vi "SetEnvTemp.vi"(11 "New temperature":dbl format="%.1f") -> (3 "Probe 1 temperature":dbl format="%.2f")   [LabVIEW 2009]
panel:
  out "error out":errorcluster
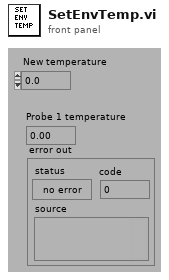
[diagram p1: front panel]
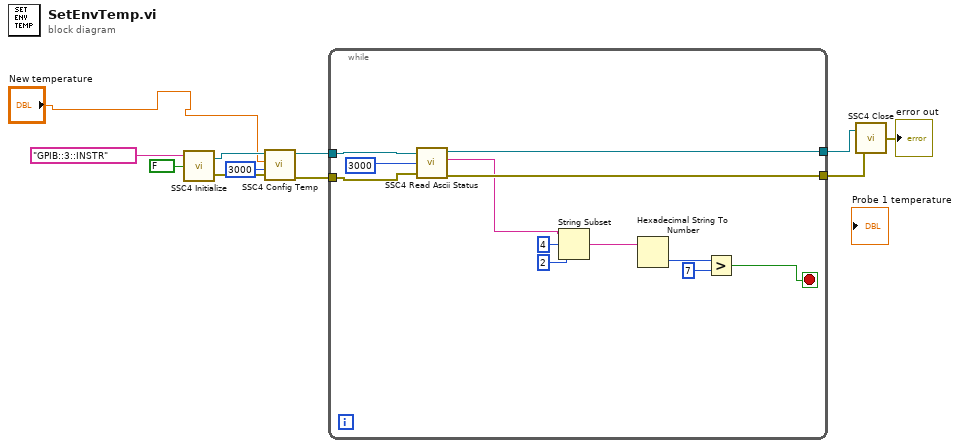
[diagram p0: block diagram]
diagram:
  n1 = call "SSC4 Initialize.vi"("reset"=FALSE, "instrument descriptor"="GPIB::3::INSTR") -> ("error out"=w8:errorcluster, "VISA session"=w9:refnum<visa-resource-name>)  [unwired: 1 in]
  n2 = call "SSC4 Config Temp.vi"("error in (no error)"=w8, "Command Delay"=u32 3000, "New temperature"="New temperature", "Visa Session"=w9) -> ("error out"=w5:errorcluster, "Dup Visa Session"=w6:refnum<visa-resource-name>)  [unwired: 6 in]
  n3 = while {
    tunnel: w6 -> [w23]
    tunnel: w5 -> [w22]
    tunnel: [w20] -> w3
    tunnel: [w19] -> w2
    stop <- w13 stop-if-true
    n4 = call "SSC4 Read Ascii Status.vi"("error in (no error)"=w22, "Command Delay (ms)"=u32 3000, "Visa Session"=w23) -> ("error out"=w19:errorcluster, "Status Byte (RSA cmd)"=w18:string, "Dup Visa Session"=w20:refnum<visa-resource-name>)  [unwired: 2 in, 1 out]
    n5 = String Subset(string=w18, offset (0)=4, length (rest)=2 ("length (rest)")) -> (substring=w15:string)
    n6 = Hexadecimal String To Number(string=w15) -> (number=w14:u32)  [unwired: 2 in, 1 out]
    n7 = Greater?(x=w14, y=u32 7) -> (0:w13:bool)
  }
  n8 = call "SSC4 Close.vi"("error in (no error)"=w2, "VISA session"=w3) -> ("error out"=→"error out":errorcluster)
